vi "StatusUpdate.vi"(8 "error in (no error)":errorcluster, 9 "Status":string, 11 "Module":refnum<class "ModuleAdmin.lvclass">) -> (0 "error out":errorcluster, 3 "Module":refnum<class "ModuleAdmin.lvclass">)   [LabVIEW 2018, in "MyPlugins.lvlib"]
uses:
  <userlib>/NIST/ModuleAdminLib/ModuleAdmin/ModuleAdmin.lvclass
  PluginsShared/clEventType.ctl
  MyPlugins/MyPlugins.lvlib
  PluginsShared/PluginsShared.lvlib
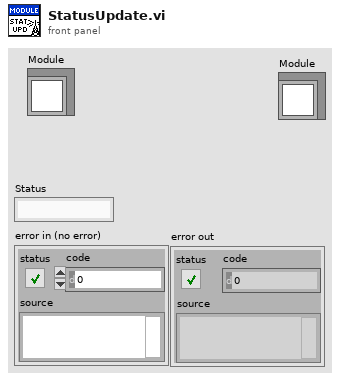
[diagram p1: front panel]
types:
  T1 = typedef "PluginsShared.lvlib/clEventType.ctl" = cluster{"ModuleID":i32, "Data":variant}
  T2 = typedef "PluginsShared.lvlib/clBroadcastEvents.ctl" = cluster{"DidInit":refnum<user-event>, "StatusUpdate":refnum<user-event>, "ErrorReport":refnum<user-event>, "DidStop":refnum<user-event>, "PathToINI":refnum<user-event>, "ReloadINIFiles":refnum<user-event>}
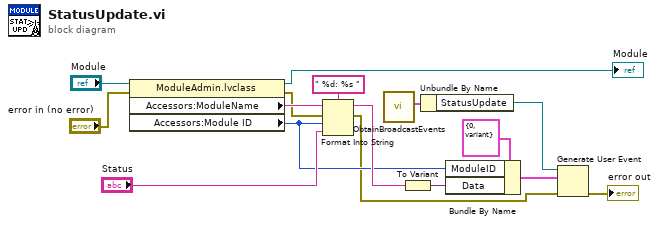
[diagram p0: block diagram]
diagram:
  n1 = property class="ModuleAdmin.lvclass"(reference="Module", error in="error in (no error)") -> (reference out=→"Module":refnum<class "ModuleAdmin.lvclass">, error out=w2:errorcluster, "Accessors:ModuleName"=w8:string, "Accessors:Module ID"=w5:i32)
  n2 = Format Into String(format string=" %d: %s ", initial string=w8, error in=w2, w5, "Status") -> (resulting string=w6:string, error out=w1:errorcluster)
  n3 = call "ObtainBroadcastEvents.vi"() -> ("clBroadcastEvents"=w16:T2)  [unwired: 10 in, 1 out]
  n4 = To Variant(anything=w6) -> (Variant=w13:variant)
  n5 = Unbundle By Name(w16) -> ("StatusUpdate"=w15:refnum<user-event>)
  n6 = Bundle By Name(cluster=T1 {"ModuleID"=0, "Data"=variant} ("clBroadcast"), "ModuleID"=w5, "Data"=w13) -> (w12:T1)
  n7 = Generate User Event(user event=w15, event data cluster=w12, error in=w1) -> (error out=→"error out":errorcluster)  [unwired: 1 in, 1 out]
